vi "FGV_CLIENT_SQL_connection.vi"(7 "options":T4, 8 "error_in":errorcluster, 9 "all_config_info_in":T1={"main_ini_file"={"SQL Driver"="", "SQL Server"="", "SQL Database"="", "SQL UID"="", "Reference table"="", "Reference history"="", "Archivisation CFG table"="", "Archivisation CFG history"="", "User table"="", "User history"="", "logout timeout [ms]"=0, "records per page"=0, "default language"="", "REF CHG connection IP"="", "REF CHG remote port"=0, "REF CHG local port"=0, "SCANNER COM port"=0, "SCANNER Baud rate"=0, "SCANNER Data bits"=0, "SCANNER Pairity"=enum."None", "SCANNER Stop bits"=10, "SCANNER Flow control"=0, "SCANNER Termination char"=0}, "SQL Password"="", "queue_refnums"={"SQL_EDITOR_queue"=refnum, "SCANNER_queue"=refnum, "SCANNER_data"=refnum, "CLIENT_REF_CHG_queue"=refnum}} {"main_ini_file"."SCANNER Flow control" items=["None"=0, "XON/XOFF"=1, "RTS/CTS"=2, "DTR/DSR"=4]; "main_ini_file"."SCANNER Stop bits" items=["1.0"=10, "1.5"=15, "2.0"=20]}, 10 "SQL_transaction":string[](array[string]), 11 "SQL_statement":string) -> (0 "error_out":errorcluster, 1 "all_config_info_out":T1={"main_ini_file"={"SQL Driver"="", "SQL Server"="", "SQL Database"="", "SQL UID"="", "Reference table"="", "Reference history"="", "Archivisation CFG table"="", "Archivisation CFG history"="", "User table"="", "User history"="", "logout timeout [ms]"=0, "records per page"=0, "default language"="", "REF CHG connection IP"="", "REF CHG remote port"=0, "REF CHG local port"=0, "SCANNER COM port"=0, "SCANNER Baud rate"=0, "SCANNER Data bits"=0, "SCANNER Pairity"=enum."None", "SCANNER Stop bits"=10, "SCANNER Flow control"=0, "SCANNER Termination char"=0}, "SQL Password"="", "queue_refnums"={"SQL_EDITOR_queue"=refnum, "SCANNER_queue"=refnum, "SCANNER_data"=refnum, "CLIENT_REF_CHG_queue"=refnum}} {"main_ini_file"."SCANNER Flow control" items=["None"=0, "XON/XOFF"=1, "RTS/CTS"=2, "DTR/DSR"=4]; "main_ini_file"."SCANNER Stop bits" items=["1.0"=10, "1.5"=15, "2.0"=20]}, 2 "connection_active?":bool, 3 "SQL_result":variant, 4 "executed_SQL_statement":string)   [LabVIEW 2019]
uses:
  FGV_CLIENT_SQL_connection.ctl
  ini/typedef/CLIENT_all_config_info.ctl
  ini/typedef/CLIENT_main_ini_file.ctl
  queues/typedef/CLIENT_queue_refnums.ctl
  queues/typedef/SQL_EDITOR_queue_element.ctl
  MAIN/SQL_EDITOR/SQL_EDITOR_sequence_state.ctl
  queues/typedef/CLIENT_SCANNER_queue_element.ctl
  MAIN/SCANNER/SCANNER_sequence_state.ctl
  queues/typedef/CLIENT_REF_CHG_queue_element.ctl
  MAIN/reference_changed_connection/CLIENT_REF_CHG_sequence_state.ctl
  <vilib>/addons/database/Auxilliary.llb/DB Tools Transaction.ctl
  <vilib>/addons/database/Connection.llb/Conn ObjectReference.ctl
  <vilib>/addons/database/Connection.llb/DB Tools Open Connec (String).vi
  <vilib>/addons/database/Connection.llb/Conn Execute.vi
  <vilib>/addons/database/Recordset.llb/Rec Destroy - Connection.vi
  <userlib>/_OpenG.lib/array/array.llb/Filter 1D Array (String)__ogtk.vi
  <vilib>/addons/database/Recordset.llb/Rec Fetch Recordset Data (R).vi
  <vilib>/addons/database/Recordset.llb/Rec Get Recordset Properties (R).vi
  <vilib>/addons/database/Recordset.llb/Rec Get Column Properties (R).vi
  <vilib>/addons/database/Connection.llb/Conn Transaction.vi
  <vilib>/addons/database/NI_Database_API.lvlib
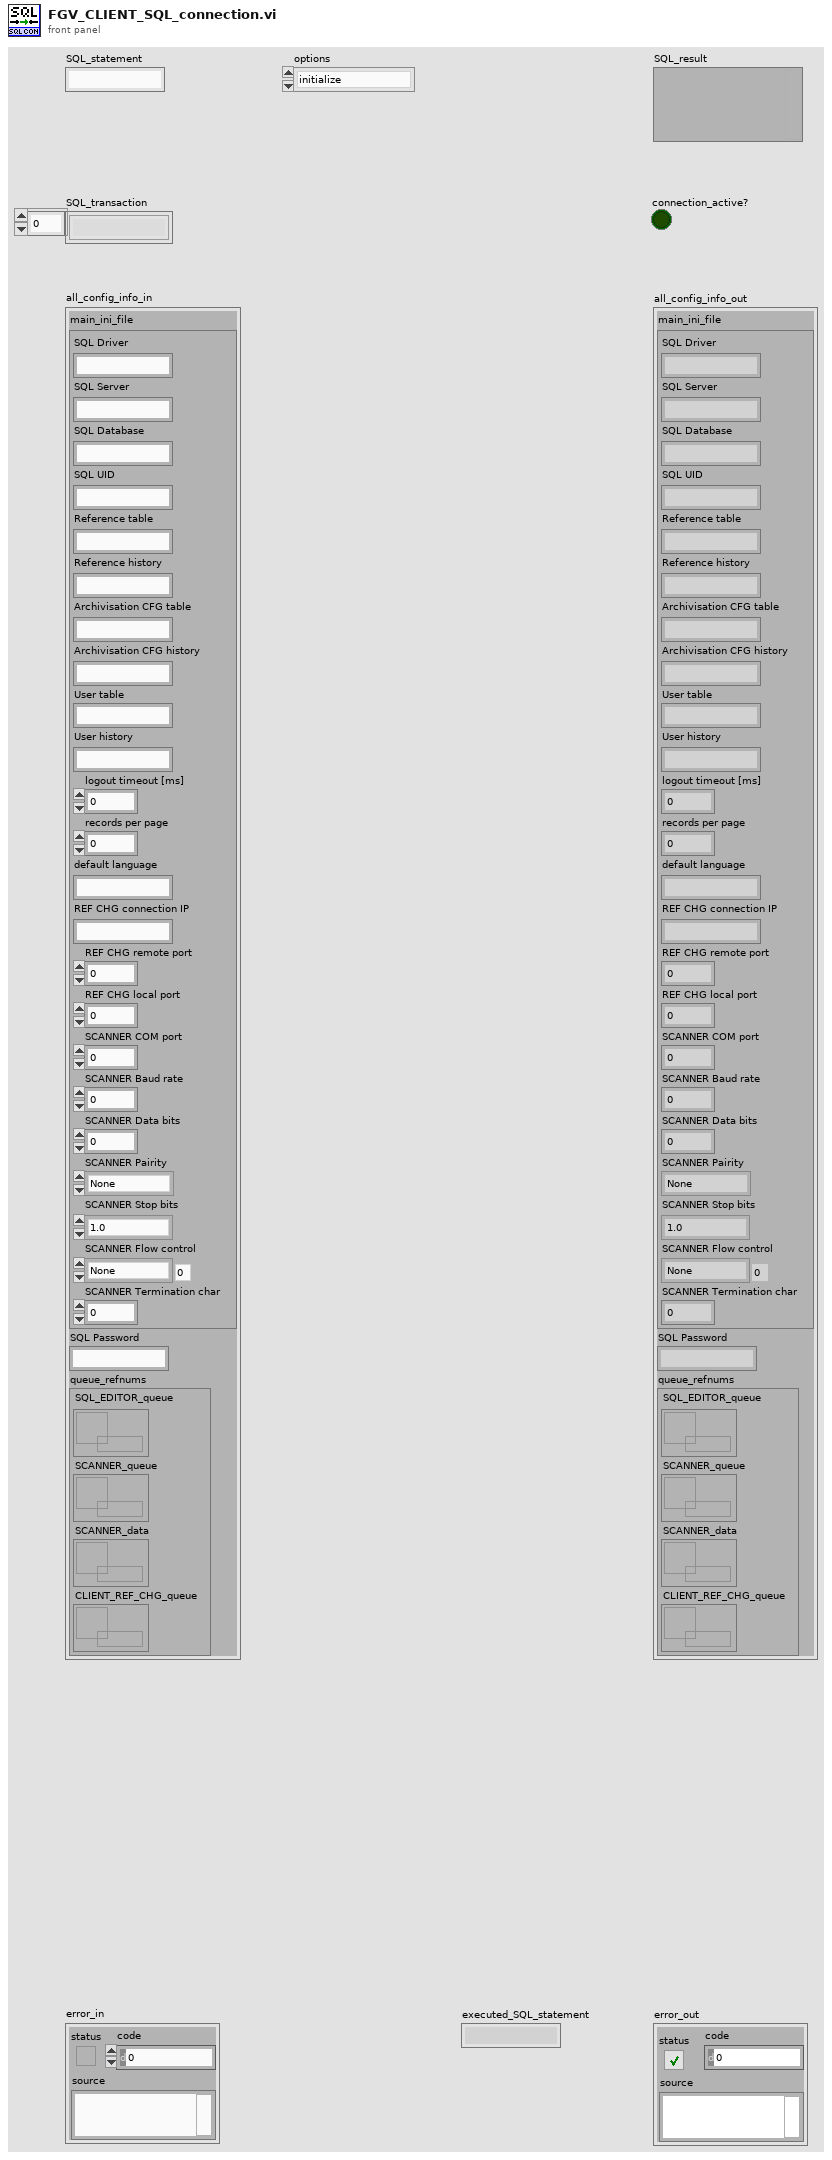
[diagram p1: front panel]
types:
  T1 = typedef "CLIENT_all_config_info.ctl" = cluster{"main_ini_file":T2, "SQL Password":string, "queue_refnums":T3}
  T2 = typedef "CLIENT_main_ini_file.ctl" = cluster{"SQL Driver":string, "SQL Server":string, "SQL Database":string, "SQL UID":string, "Reference table":string, "Reference history":string, "Archivisation CFG table":string, "Archivisation CFG history":string, "User table":string, "User history":string, "logout timeout [ms]":i32, "records per page":i32, "default language":string, "REF CHG connection IP":string, "REF CHG remote port":i32, "REF CHG local port":i32, "SCANNER COM port":u16, "SCANNER Baud rate":u32, "SCANNER Data bits":u16, "SCANNER Pairity":enum16{"None", "Odd", "Even", "Mark", "Space"}, "SCANNER Stop bits":u16, "SCANNER Flow control":u16, "SCANNER Termination char":u8}
  T3 = typedef "CLIENT_queue_refnums.ctl" = cluster{"SQL_EDITOR_queue":refnum<queue>, "SCANNER_queue":refnum<queue>, "SCANNER_data":refnum<queue>, "CLIENT_REF_CHG_queue":refnum<queue>}
  T4 = typedef "FGV_CLIENT_SQL_connection.ctl" = enum16{"initialize", "connect", "read_tables", "read_columns", "SELECT", "INSERT", "UPDATE", "DELETE", "EXEC + headers", "EXEC", "TRANSACTION", "connection_active?", "disconnect"}
  T5 = typedef "NI_Database_API.lvlib/DB Tools Transaction.ctl" = enum16{"begin", "commit", "rollback"}
  T6 = typedef "NI_Database_API.lvlib/Conn ObjectReference.ctl" = refnum<k1>
  T7 = typedef "NI_Database_API.lvlib/Rec ObjectReference.ctl" = refnum<k1>
  T8 = typedef "NI_Database_API.lvlib/Rec Properties.ctl" = cluster{"column count":i32, "record index":i32, "record count":i32, "bof?":bool, "eof?":bool, "cursor type":T9, "cache size":i32, "state":enum16{"closed", "open"}}
  T9 = typedef "NI_Database_API.lvlib/DB Tools Cursor Type.ctl" = enum16{"forward-only", "keyset", "dynamic", "static"}
  T10 = typedef "NI_Database_API.lvlib/Rec Column Properties.ctl" = cluster{"name":string, "database data type":T11, "defined size":i32, "actual size":i32}
  T11 = typedef "NI_Database_API.lvlib/DB Tools DataTypes.ctl" = enum16{"String", "Long (I32)", "Single (SGL)", "Double (DBL)", "Date/Time", "Binary"}
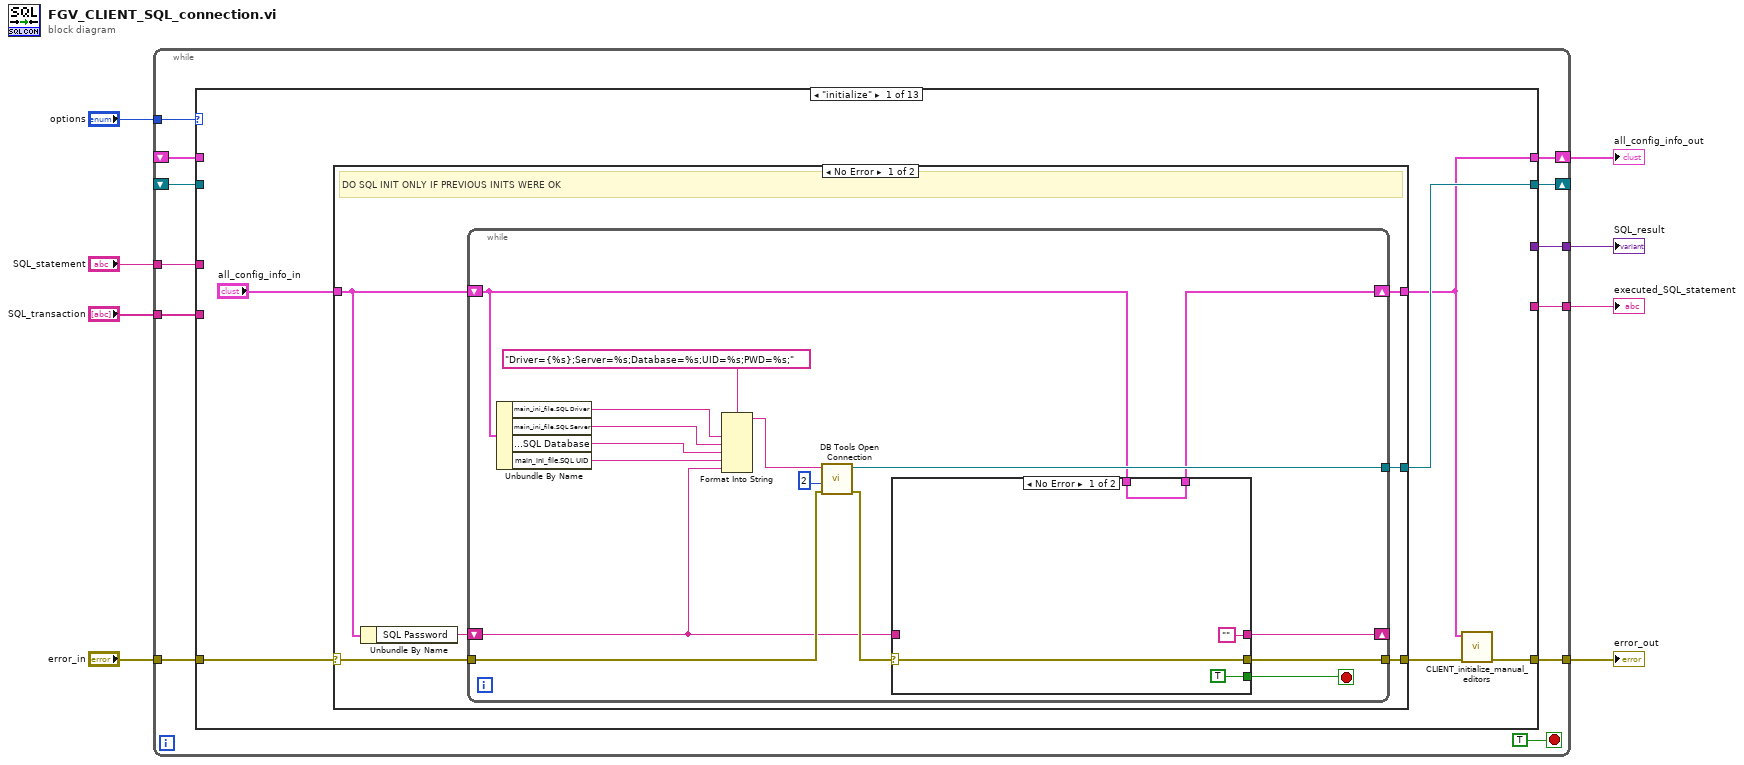
[diagram p0: block diagram]
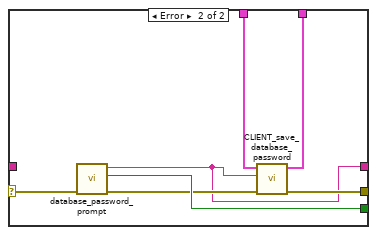
[diagram p2: hidden frame]
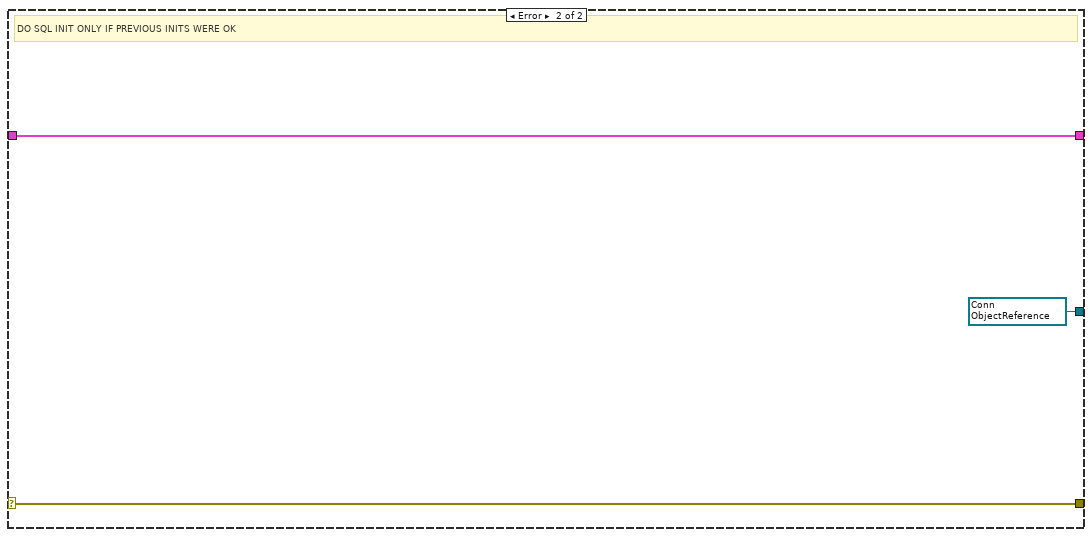
[diagram p3: hidden frame]
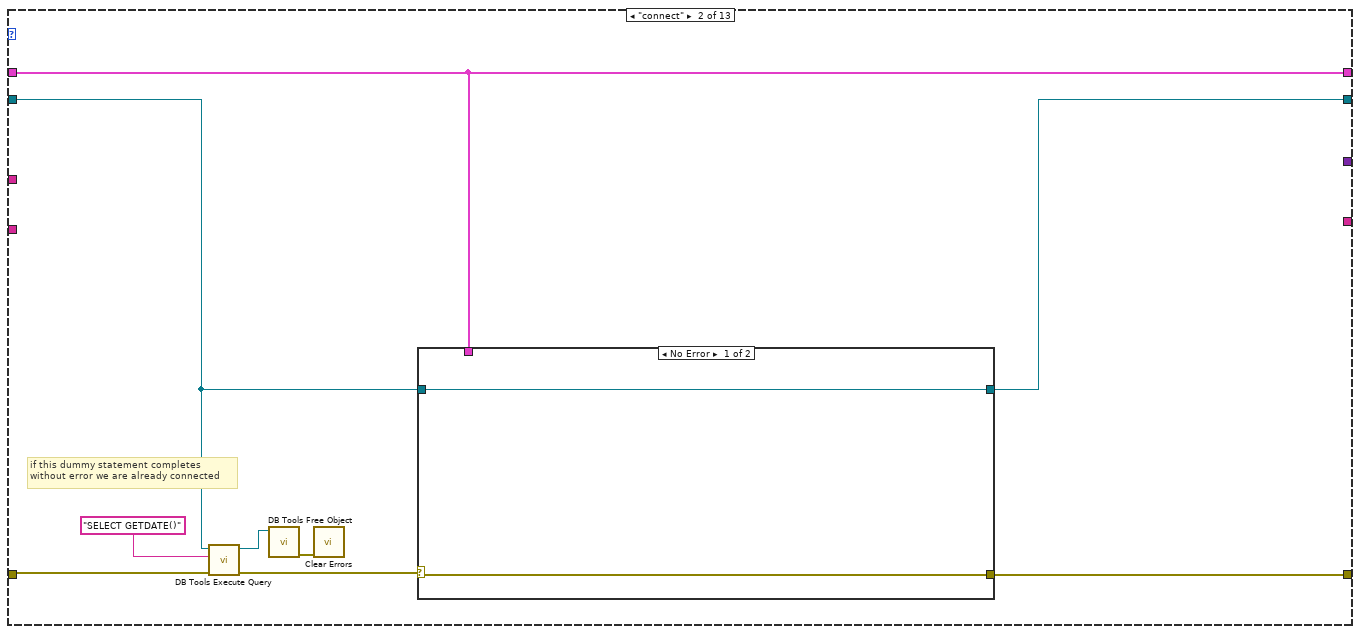
[diagram p4: hidden frame]
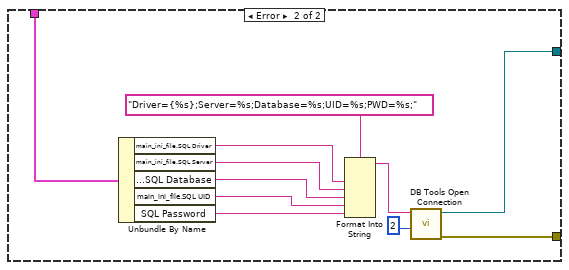
[diagram p5: hidden frame]
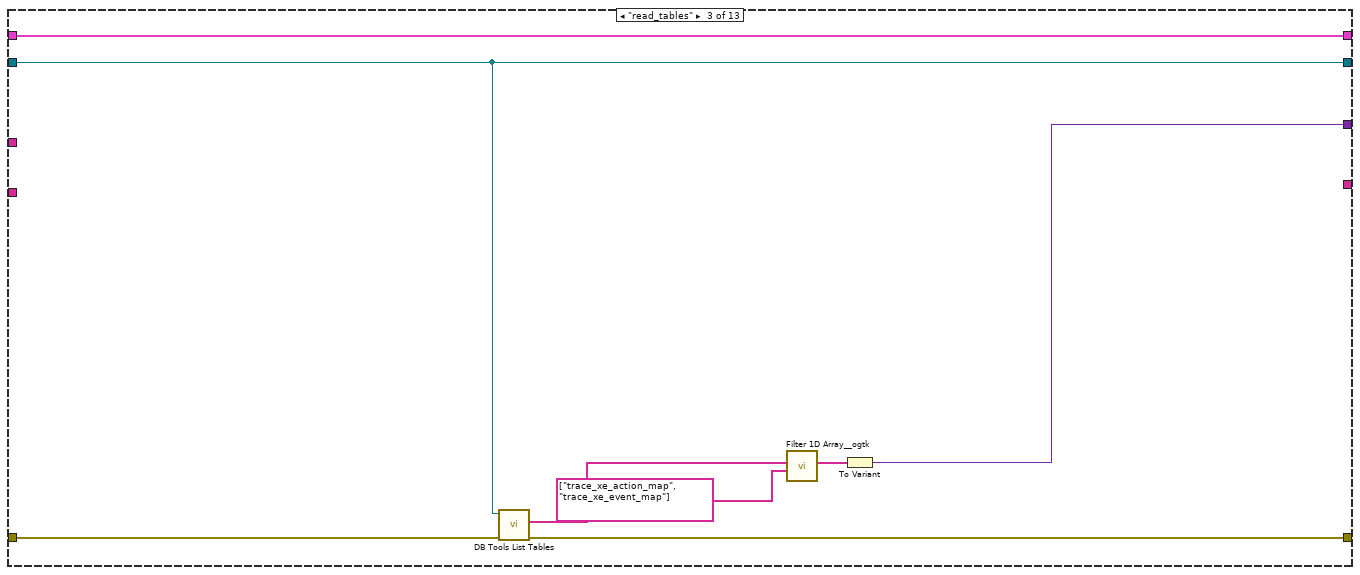
[diagram p6: hidden frame]
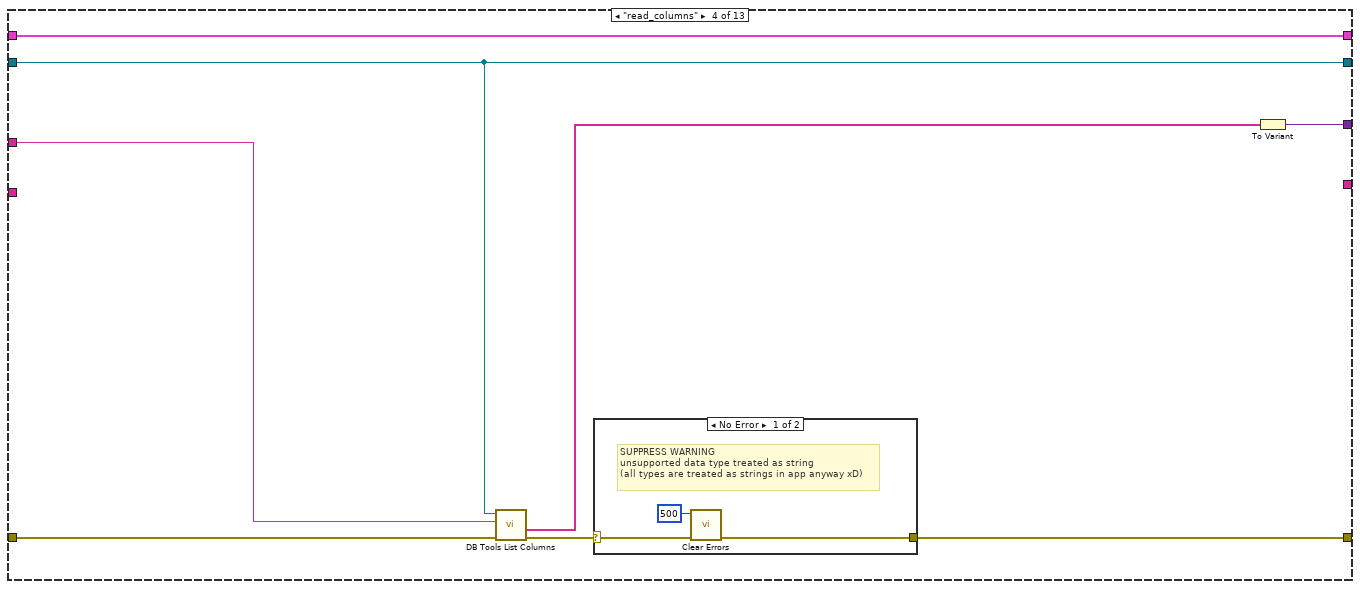
[diagram p7: hidden frame]
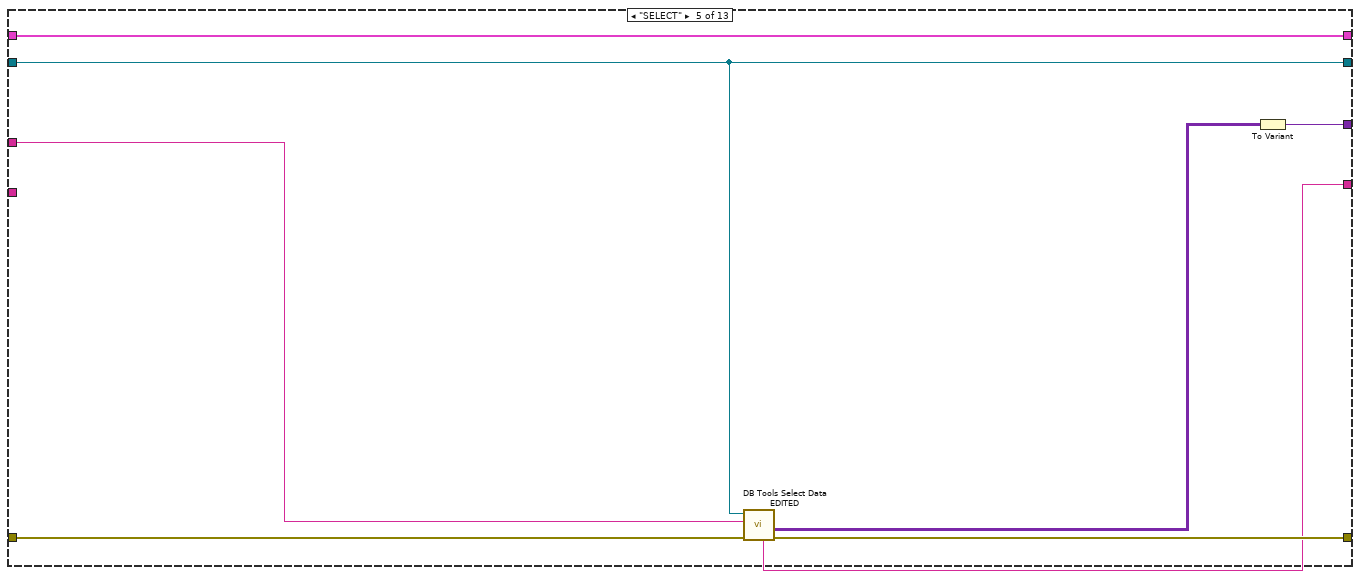
[diagram p9: hidden frame]
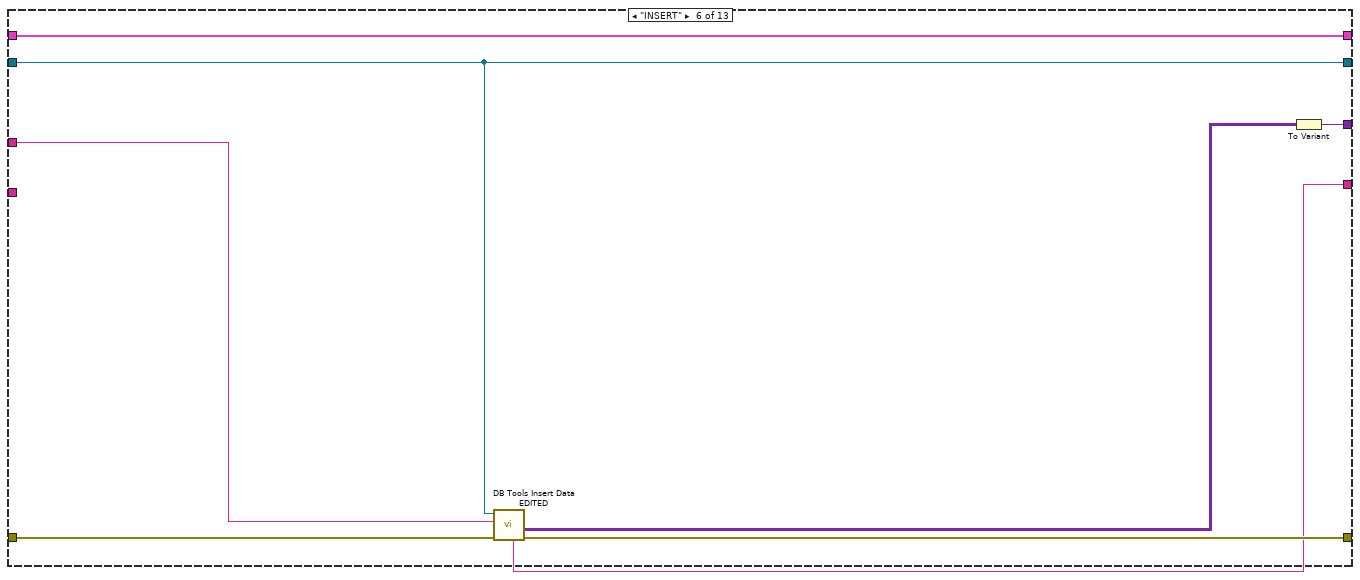
[diagram p10: hidden frame]
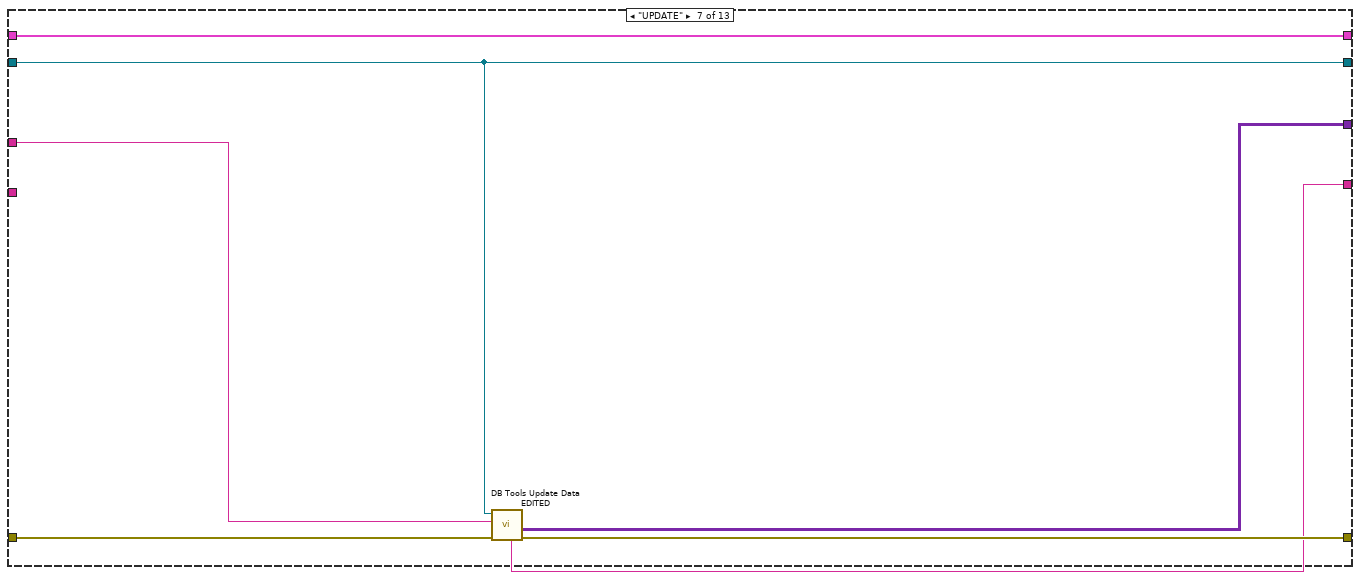
[diagram p11: hidden frame]
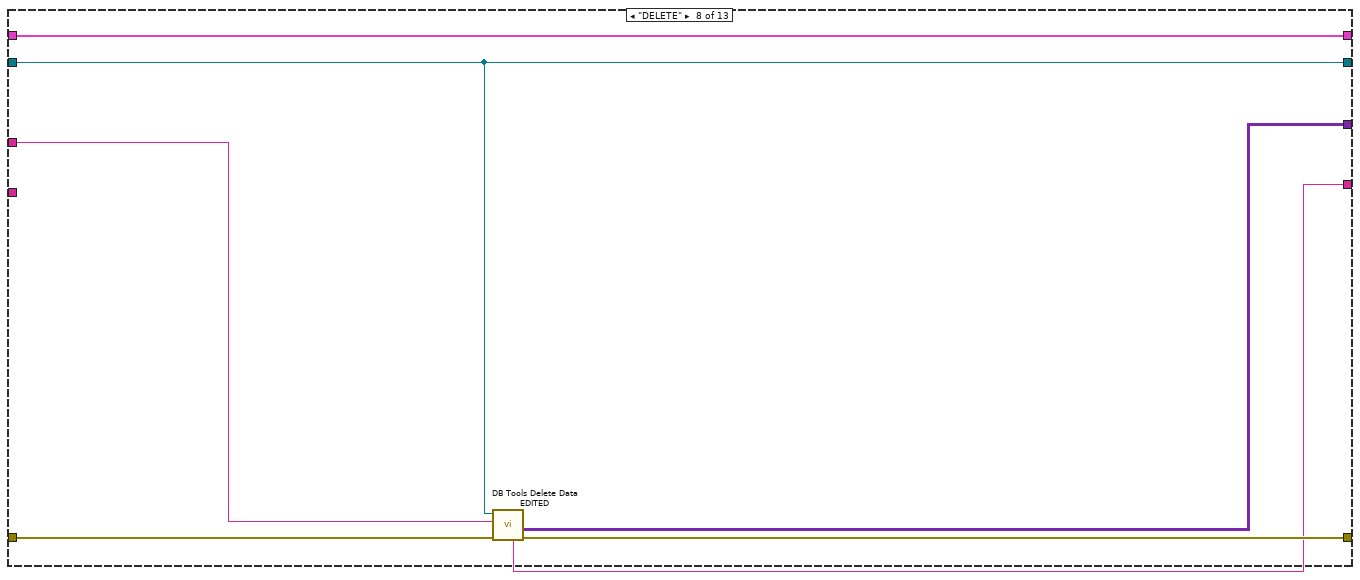
[diagram p12: hidden frame]
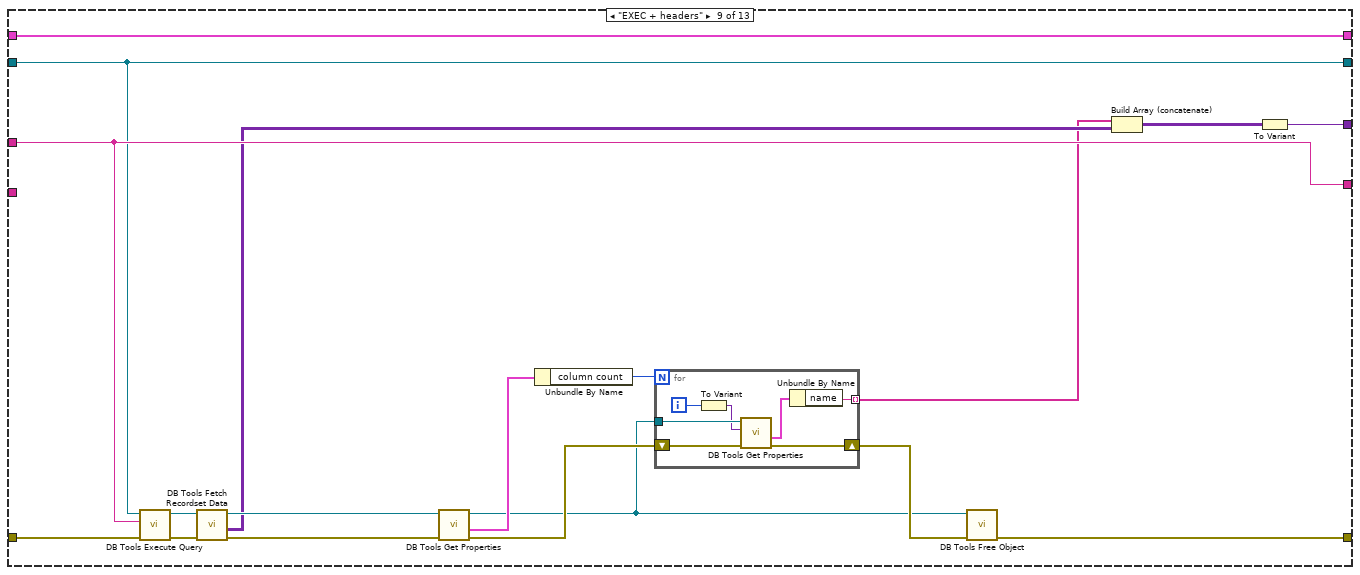
[diagram p13: hidden frame]
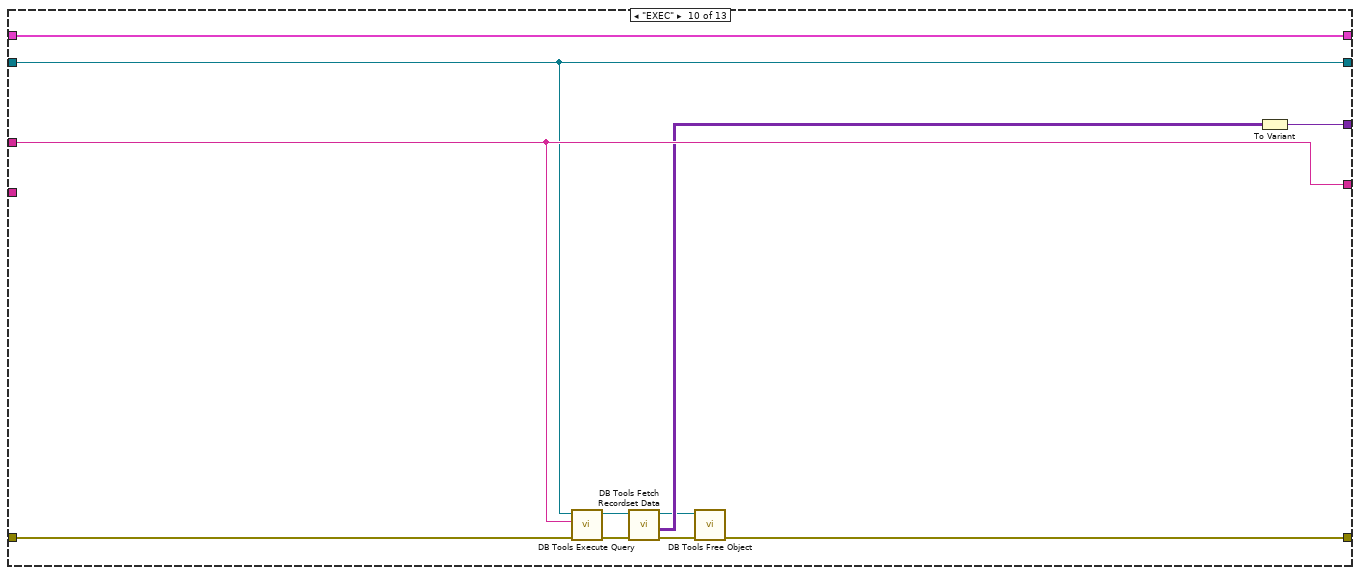
[diagram p14: hidden frame]
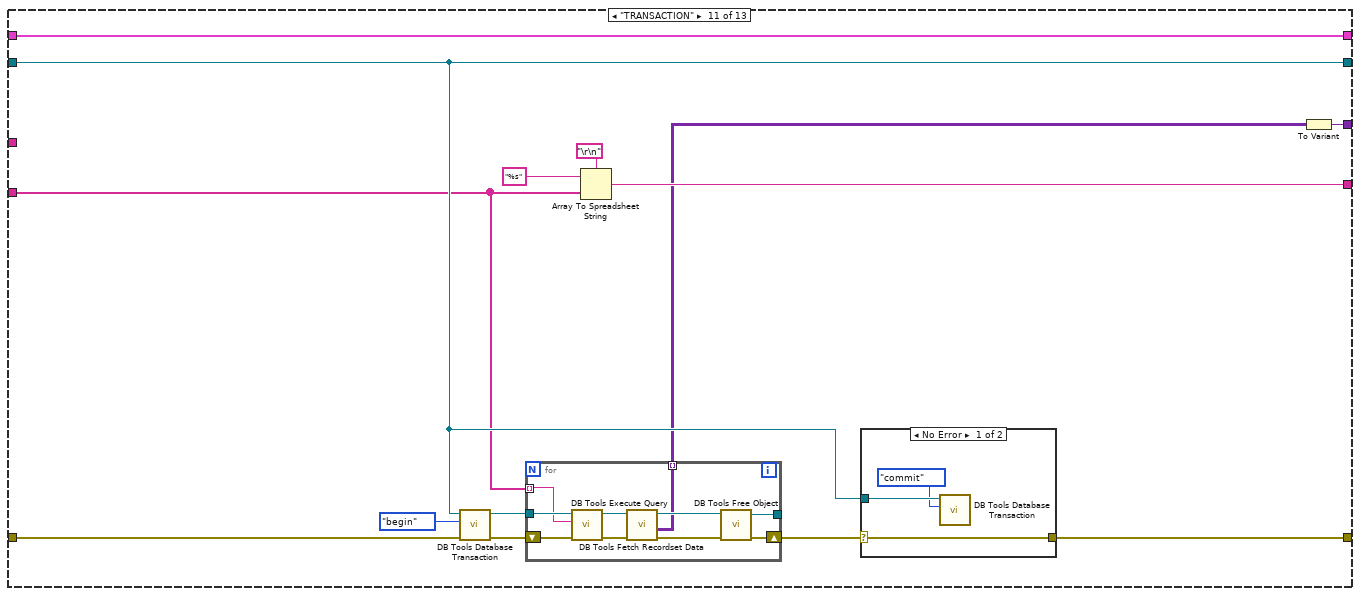
[diagram p15: hidden frame]
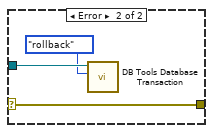
[diagram p16: hidden frame]
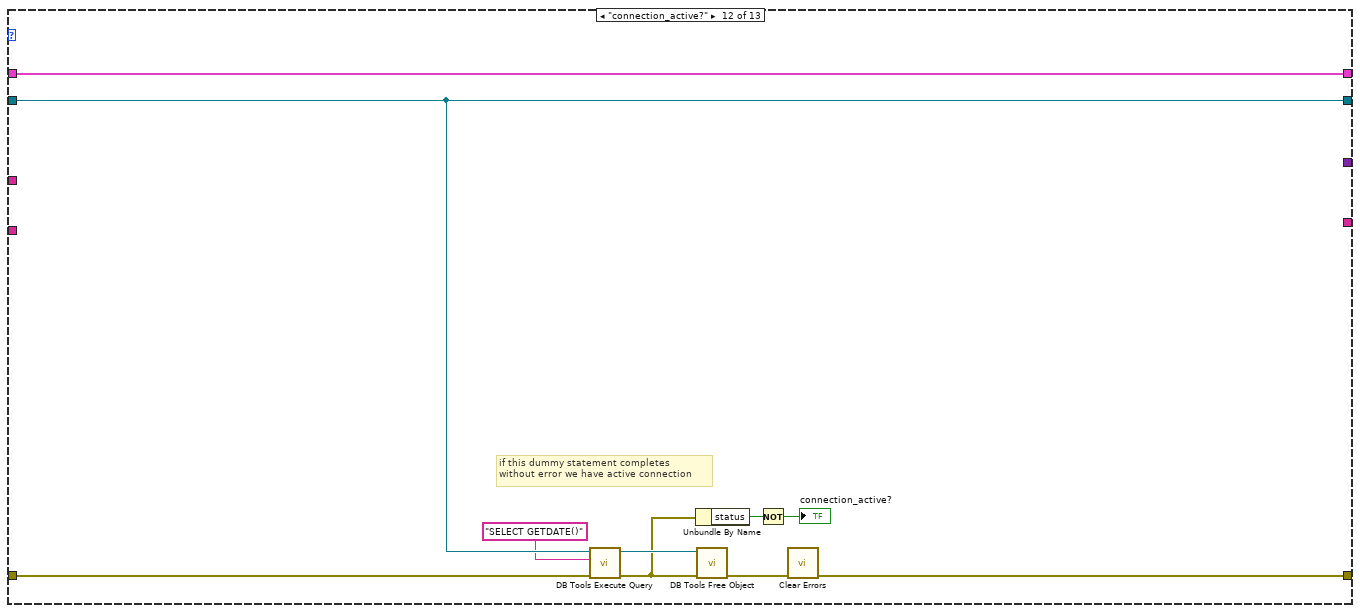
[diagram p17: hidden frame]
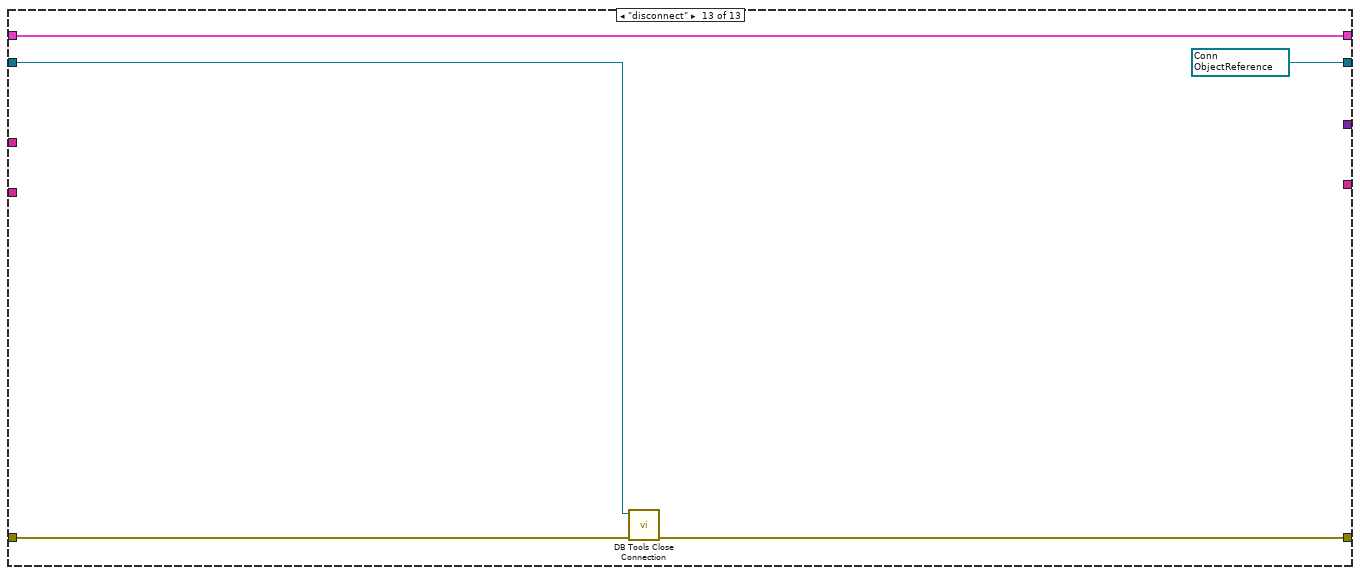
[diagram p18: hidden frame]
diagram:
  n1 = while {
    tunnel: "options" -> [w19]
    tunnel: [w18] -> w8
    tunnel: "error_in" -> [w17]
    shift-right: [w15] -> w1
    shift-left: _ -> [w16]
    shift-right: [w14] -> _
    shift-left: _ -> [w13]
    tunnel: [w12] -> w5
    tunnel: "SQL_statement" -> [w11]
    tunnel: [w10] -> w3
    tunnel: "SQL_transaction" -> [w9]
    stop <- TRUE stop-if-true
    n2 = case shown="\"initialize\"" w19 {
      tunnel: [w24 w69 w87 w93 w109 w119 w125 w133 w148 w166 w178 w206 w211] -> w18
      tunnel: w17 -> [w25 w67 w88 w99 w110 w118 w126 w132 w149 w167 w181 w210 w212]
      tunnel: w16 -> [_ w70 w92 w100 w106 w120 w127 w134 w152 w170 w184 w209 w215]
      tunnel: [w21 w70 w92 w100 w106 w120 w127 w134 w152 w170 w184 w209 w215] -> w15
      tunnel: [w26 w71 w85 w98 w111 w116 w123 w129 w146 w164 w177 w208 w213] -> w14
      tunnel: w13 -> [_ w65 w85 w98 w111 w116 w123 w129 w146 w164 w177 w208 w214]
      tunnel: [_ _ w86 w97 w112 w114 w121 w128 w145 w163 w172 _ _] -> w12
      tunnel: w11 -> [_ _ _ w95 w105 w117 w122 w130 w147 w165 _ _ _]
      tunnel: [_ _ _ _ w107 w115 w124 w131 w147 w165 w175 _ _] -> w10
      tunnel: w9 -> [_ _ _ _ _ _ _ _ _ _ w176 _ _]
      frame "initialize" {
        n3 = case shown="No Error" w25 {
          selector: w25 -> [w31 w60]
          tunnel: [w32 w62] -> w26
          tunnel: "all_config_info_in" -> [w29 w61]
          tunnel: [w28 w60] -> w22
          tunnel: [w27 w61] -> w21
          frame No Error {
            # "DO SQL INIT ONLY IF PREVIOUS INITS WERE OK"
            n4 = Unbundle By Name(w29) -> ("SQL Password"=w30:string)
            n5 = while {
              tunnel: [w43] -> w32
              shift-right: [w36] -> _
              shift-left: w30 -> [w37]
              tunnel: w31 -> [w41]
              tunnel: [w35] -> w28
              shift-right: [w34] -> w27
              shift-left: w29 -> [w33]
              stop <- w39 stop-if-true
              n6 = Unbundle By Name(w33) -> ("main_ini_file.SQL Driver"=w46:string, "main_ini_file.SQL Server"=w45:string, "main_ini_file.SQL Database"=w44:string, "main_ini_file.SQL UID"=w38:string)
              n7 = Format Into String(format string="Driver={%s};Server=%s;Database=%s;UID=%s;PWD=%s;", w46, w45, w44, w38, w37) -> (resulting string=w48:string)  [unwired: 2 in, 1 out]
              n8 = call-poly <vilib>:"DB Tools Open Connection.vi"("error in (no error)"=w41, "connection timeout (15)"=2, "connection information"=w48) -> ("error out"=w40:errorcluster, "connection reference"=w43:T6)  [unwired: 5 in]
              n9 = case shown="No Error" w40 {
                selector: w40 -> [w52 w59]
                tunnel: [w52 w54] -> w35
                tunnel: [TRUE w58] -> w39
                tunnel: w37 -> [_ _]
                tunnel: w33 -> [w50 w56]
                tunnel: [w50 w55] -> w34
                tunnel: ["" w53] -> w36
                frame No Error {
                }
                frame Error {
                  n10 = call "database_password_prompt.vi"("error_in"=w59) -> ("error_out"=w57:errorcluster, "Canceled?"=w58:bool, "new_password"=w53:string)  [unwired: 8 in]
                  n11 = call "CLIENT_save_database_password.vi"("error_in"=w57, "new_password"=w53, "all_config_info_in"=w56) -> ("error_out"=w54:errorcluster, "all_config_info_out"=w55:T1)  [unwired: 6 in]
                }
              }
            }
          }
          frame Error {
            w62 = T6 refnum items=["Connection"] ("connection reference")
            # "DO SQL INIT ONLY IF PREVIOUS INITS WERE OK"
          }
        }
        n12 = call "CLIENT_initialize_manual_editors.vi"("error_in"=w22, "all_config_info"=w21) -> ("error_out"=w24:errorcluster)  [unwired: 9 in]
      }
      frame "connect" {
        # "if this dummy statement completes\nwithout error we are already connected"
        n13 = call-poly <vilib>:"DB Tools Execute Query.vi"("error in (no error)"=w67, "SQL query"="SELECT GETDATE()", "connection reference"=w65) -> ("error out"=w64:errorcluster, "recordset reference"=w66:T7)  [unwired: 5 in]
        n14 = call-poly <vilib>:"DB Tools Free Object.vi"("recordset reference"=w66) -> ("error out"=w63:errorcluster)  [unwired: 9 in, 1 out]
        n15 = call <vilib>:"Clear Errors.vi"("error in (no error)"=w63) -> ()  [unwired: 5 in, 2 out]
        n16 = case shown="No Error" w64 {
          selector: w64 -> [w72 _]
          tunnel: [w73 w77] -> w71
          tunnel: w70 -> [_ w76]
          tunnel: [w72 w74] -> w69
          tunnel: w65 -> [w73 _]
          frame No Error {
          }
          frame Error {
            n17 = Unbundle By Name(w76) -> ("main_ini_file.SQL Driver"=w82:string, "main_ini_file.SQL Server"=w81:string, "main_ini_file.SQL Database"=w80:string, "main_ini_file.SQL UID"=w79:string, "SQL Password"=w78:string)
            n18 = Format Into String(format string="Driver={%s};Server=%s;Database=%s;UID=%s;PWD=%s;", w82, w81, w80, w79, w78) -> (resulting string=w84:string)  [unwired: 2 in, 1 out]
            n19 = call-poly <vilib>:"DB Tools Open Connection.vi"("connection timeout (15)"=2, "connection information"=w84) -> ("error out"=w74:errorcluster, "connection reference"=w77:T6)  [unwired: 6 in]
          }
        }
      }
      frame "read_tables" {
        n20 = call <vilib>:"DB Tools List Tables.vi"("error in (no error)"=w88, "connection reference"=w85) -> ("error out"=w87:errorcluster, "tables"=w91:string[])  [unwired: 3 in, 1 out]
        n21 = call-poly <userlib>:"Filter 1D Array__ogtk.vi"("items to filter"=string[] ["trace_xe_action_map", "trace_xe_event_map"], "array"=w91) -> ("filtered array"=w89:string[])  [unwired: 4 in, 1 out]
        n22 = To Variant(anything=w89) -> (Variant=w86:variant)
      }
      frame "read_columns" {
        n23 = call <vilib>:"DB Tools List Columns.vi"("error in (no error)"=w99, "table"=w95, "connection reference"=w98) -> ("error out"=w94:errorcluster, "columns"=w96:string[])  [unwired: 1 in, 2 out]
        n24 = case shown="No Error" w94 {
          selector: w94 -> [w103 w104]
          tunnel: [w102 w104] -> w93
          frame No Error {
            # "SUPPRESS WARNING\nunsupported data type treated as string\n(all types are treated as strings in app anyway xD)"
            n25 = call <vilib>:"Clear Errors.vi"("error in (no error)"=w103, "specific error code to clear (0: all)"=500) -> ("error out"=w102:errorcluster)  [unwired: 4 in, 1 out]
          }
          frame Error {
          }
        }
        n26 = To Variant(anything=w96) -> (Variant=w97:variant)
      }
      frame "SELECT" {
        n27 = call "DB Tools Select Data EDITED.vi"("error_in"=w110, "SELECT_statement"=w105, "connection_reference_in"=w111) -> ("error_out"=w109:errorcluster, "SQL_result"=w108:variant[][], "executed_SQL_statement"=w107:string)  [unwired: 5 in, 1 out]
        n28 = To Variant(anything=w108) -> (Variant=w112:variant)
      }
      frame "INSERT" {
        n29 = call "DB Tools Insert Data EDITED.vi"("error_in"=w118, "INSERT_statement"=w117, "connection_reference_in"=w116) -> ("error_out"=w119:errorcluster, "SQL_result"=w113:variant[][], "executed_SQL_statement"=w115:string)  [unwired: 5 in, 1 out]
        n30 = To Variant(anything=w113) -> (Variant=w114:variant)
      }
      frame "UPDATE" {
        n31 = call "DB Tools Update Data EDITED.vi"("error_in"=w126, "UPDATE_statement"=w122, "connection_reference_in"=w123) -> ("error_out"=w125:errorcluster, "SQL_result"=w121:variant[][], "executed_SQL_statement"=w124:string)  [unwired: 5 in, 1 out]
      }
      frame "DELETE" {
        n32 = call "DB Tools Delete Data EDITED.vi"("error_in"=w132, "UPDATE_statement"=w130, "connection_reference_in"=w129) -> ("error_out"=w133:errorcluster, "SQL_result"=w128:variant[][], "executed_SQL_statement"=w131:string)  [unwired: 5 in, 1 out]
      }
      frame "EXEC + headers" {
        n33 = call-poly <vilib>:"DB Tools Execute Query.vi"("error in (no error)"=w149, "SQL query"=w147, "connection reference"=w146) -> ("error out"=w151:errorcluster, "recordset reference"=w150:T7)  [unwired: 5 in]
        n34 = call-poly <vilib>:"DB Tools Fetch Recordset Data.vi"("error in (no error)"=w151, "recordset reference"=w150) -> ("error out"=w141:errorcluster, "recordset data"=w137:variant[][], "recordset reference out"=w139:T7)  [unwired: 3 in]
        n35 = call-poly <vilib>:"DB Tools Get Properties.vi"("error in (no error)"=w141, "recordset reference"=w139) -> ("error out"=w143:errorcluster, "recordset properties"=w142:T8, "recordset reference out"=w138:T7)  [unwired: 3 in]
        n36 = Unbundle By Name(w142) -> ("column count"=w144:i32)
        n37 = for {
          N: w144 -> [_]
          tunnel: w138 -> [w159]
          tunnel: [w155] -> w135 mode=indexing
          shift-right: [w153] -> w140
          shift-left: w143 -> [w154]
          i -> [w157]
          n38 = To Variant(anything=w157) -> (Variant=w158:variant)
          n39 = call-poly <vilib>:"DB Tools Get Properties.vi"("error in (no error)"=w154, "column index"=w158, "recordset reference"=w159) -> ("error out"=w153:errorcluster, "column properties"=w156:T10)  [unwired: 2 in, 1 out]
          n40 = Unbundle By Name(w156) -> ("name"=w155:string)
        }
        n41 = call-poly <vilib>:"DB Tools Free Object.vi"("error in (no error)"=w140, "recordset reference"=w138) -> ("error out"=w148:errorcluster)  [unwired: 8 in, 1 out]
        n42 = Build Array (concatenate)(w135, w137) -> (w136:variant[][])
        n43 = To Variant(anything=w136) -> (Variant=w145:variant)
      }
      frame "EXEC" {
        n44 = call-poly <vilib>:"DB Tools Execute Query.vi"("error in (no error)"=w167, "SQL query"=w165, "connection reference"=w164) -> ("error out"=w169:errorcluster, "recordset reference"=w168:T7)  [unwired: 5 in]
        n45 = call-poly <vilib>:"DB Tools Fetch Recordset Data.vi"("error in (no error)"=w169, "recordset reference"=w168) -> ("error out"=w160:errorcluster, "recordset data"=w162:variant[][], "recordset reference out"=w161:T7)  [unwired: 3 in]
        n46 = call-poly <vilib>:"DB Tools Free Object.vi"("error in (no error)"=w160, "recordset reference"=w161) -> ("error out"=w166:errorcluster)  [unwired: 8 in, 1 out]
        n47 = To Variant(anything=w162) -> (Variant=w163:variant)
      }
      frame "TRANSACTION" {
        n48 = call-poly <vilib>:"DB Tools Database Transaction.vi"("error in (no error)"=w181, "operation (begin)"=DB_Tools_Transaction."begin", "connection reference"=w177) -> ("error out"=w182:errorcluster, "connection reference out"=w180:T6)  [unwired: 3 in]
        n49 = for {
          tunnel: w180 -> [w193]
          tunnel: [w191] -> _
          shift-right: [w192] -> w179
          shift-left: w182 -> [w194]
          tunnel: w176 -> [w190] mode=indexing
          tunnel: [w185] -> w171 mode=indexing
          n50 = call-poly <vilib>:"DB Tools Execute Query.vi"("error in (no error)"=w194, "SQL query"=w190, "connection reference"=w193) -> ("error out"=w186:errorcluster, "recordset reference"=w189:T7)  [unwired: 5 in]
          n51 = call-poly <vilib>:"DB Tools Fetch Recordset Data.vi"("error in (no error)"=w186, "recordset reference"=w189) -> ("error out"=w187:errorcluster, "recordset data"=w185:variant[][], "recordset reference out"=w188:T7)  [unwired: 3 in]
          n52 = call-poly <vilib>:"DB Tools Free Object.vi"("error in (no error)"=w187, "recordset reference"=w188) -> ("error out"=w192:errorcluster, "connection reference"=w191:T6)  [unwired: 8 in]
        }
        n53 = Array To Spreadsheet String(delimiter (Tab)="\r\n", array=w176, 3:"%s" ("format string")) -> (spreadsheet string=w175:string)
        n54 = case shown="No Error" w179 {
          selector: w179 -> [w195 w198]
          tunnel: w177 -> [w197 w200]
          tunnel: [w195 w198] -> w178
          frame No Error {
            n55 = call-poly <vilib>:"DB Tools Database Transaction.vi"("operation (begin)"=DB_Tools_Transaction."commit", "connection reference"=w197) -> ()  [unwired: 4 in, 2 out]
          }
          frame Error {
            n56 = call-poly <vilib>:"DB Tools Database Transaction.vi"("operation (begin)"=DB_Tools_Transaction."rollback", "connection reference"=w200) -> ()  [unwired: 4 in, 2 out]
          }
        }
        n57 = To Variant(anything=w171) -> (Variant=w172:variant)
      }
      frame "connection_active?" {
        # "if this dummy statement completes\nwithout error we have active connection"
        n58 = call-poly <vilib>:"DB Tools Execute Query.vi"("error in (no error)"=w210, "SQL query"="SELECT GETDATE()", "connection reference"=w208) -> ("error out"=w203:errorcluster, "recordset reference"=w205:T7)  [unwired: 5 in]
        n59 = Unbundle By Name(w203) -> ("status"=w202:bool)
        n60 = call-poly <vilib>:"DB Tools Free Object.vi"("error in (no error)"=w203, "recordset reference"=w205) -> ("error out"=w204:errorcluster)  [unwired: 8 in, 1 out]
        n61 = Not(x=w202) -> (.not. x?=→"connection_active?":bool)
        n62 = call <vilib>:"Clear Errors.vi"("error in (no error)"=w204) -> ("error out"=w206:errorcluster)  [unwired: 5 in, 1 out]
      }
      frame "disconnect" {
        w213 = T6 refnum items=["Connection"] ("connection reference")
        n63 = call <vilib>:"DB Tools Close Connection.vi"("error in (no error)"=w212, "connection reference"=w214) -> ("error out"=w211:errorcluster)  [unwired: 5 in]
      }
    }
  }
  "error_out" <- w8
  "SQL_result" <- w5
  "executed_SQL_statement" <- w3
  "all_config_info_out" <- w1
